vi "7_segment.vi"() -> ()   [LabVIEW 2019]
panel:
  in  "Numeric":i32
  out "F":bool
  out "E":bool
  out "C":bool
  out "B":bool
  out "D":bool
  out "G":bool
  out "A":bool
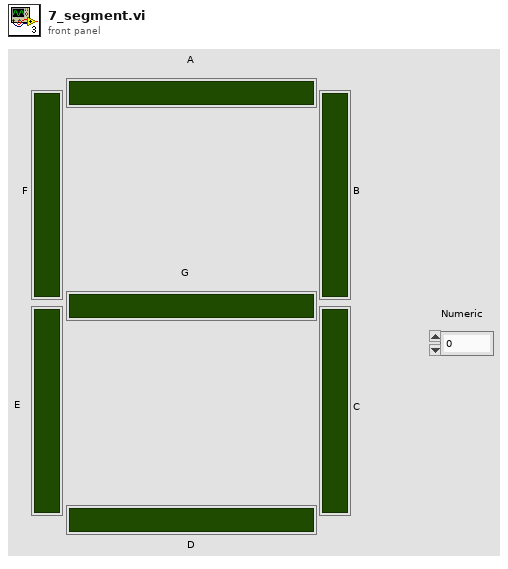
[diagram p1: front panel]
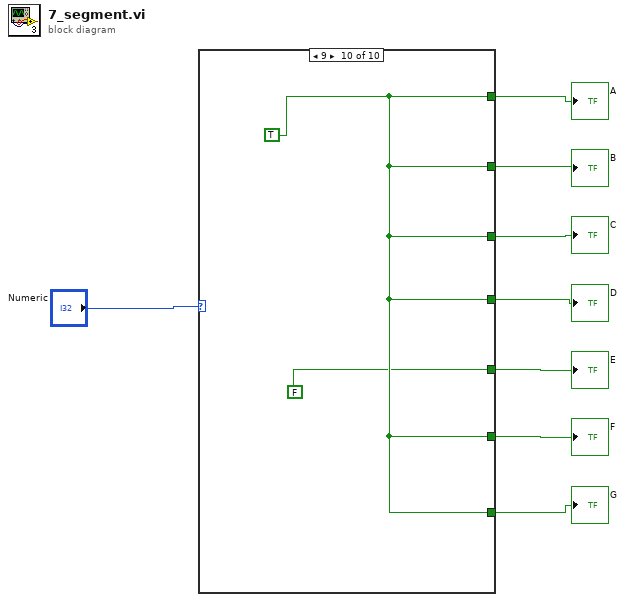
[diagram p0: block diagram]
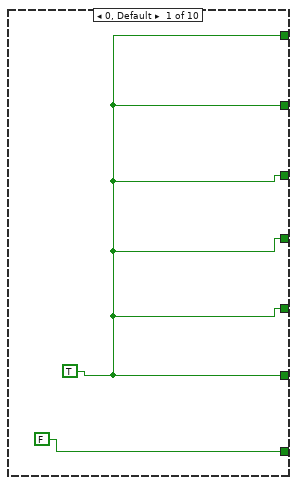
[diagram p2: hidden frame]
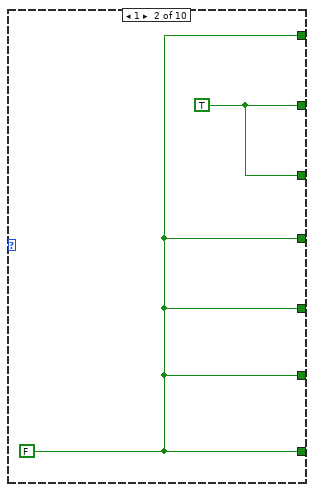
[diagram p3: hidden frame]
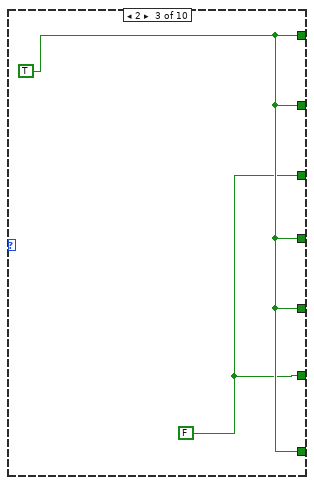
[diagram p4: hidden frame]
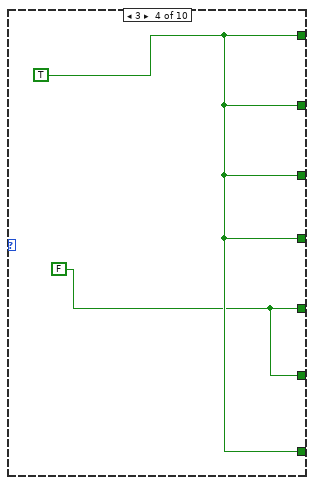
[diagram p5: hidden frame]
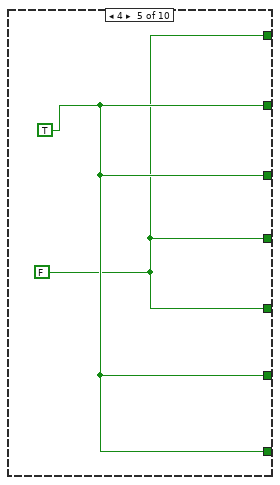
[diagram p6: hidden frame]
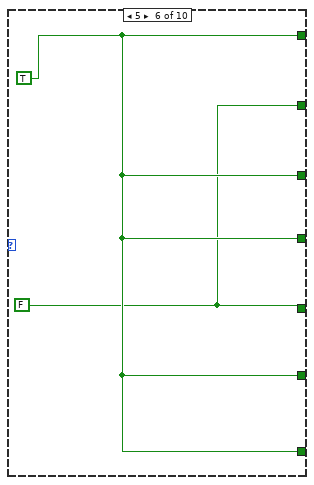
[diagram p7: hidden frame]
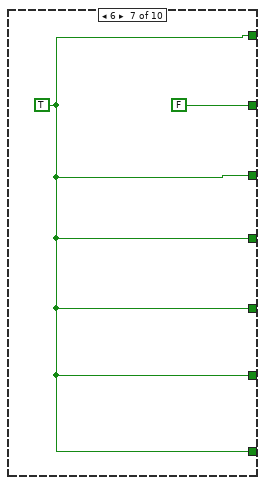
[diagram p8: hidden frame]
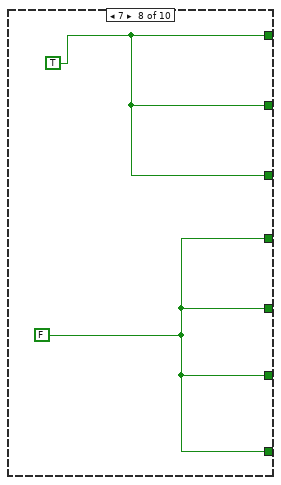
[diagram p9: hidden frame]
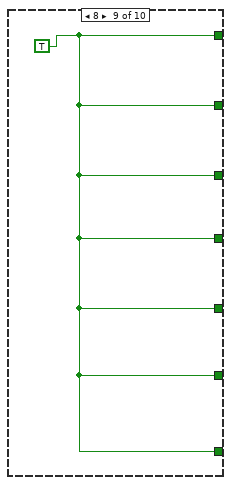
[diagram p10: hidden frame]
diagram:
  n1 = case shown="9" "Numeric" {
    tunnel: [w10 w11 w14 w16 w17 w20 w21 w24 w25 w27] -> w7
    tunnel: [w10 w12 w14 w16 w18 w19 FALSE w24 w25 w27] -> w6
    tunnel: [w10 w12 w13 w16 w18 w20 w21 w24 w25 w27] -> w5
    tunnel: [FALSE w11 w14 w16 w18 w20 w21 w23 w25 w27] -> w4
    tunnel: [w10 w11 w13 w15 w18 w20 w21 w23 w25 w27] -> w3
    tunnel: [w10 w11 w14 w15 w17 w19 w21 w23 w25 FALSE] -> w2
    tunnel: [w10 w11 w14 w16 w17 w20 w21 w23 w25 w27] -> w1
    frame 0, Default {
      w10 = TRUE
    }
    frame 1 {
      w12 = TRUE
      w11 = FALSE
    }
    frame 2 {
      w13 = FALSE
      w14 = TRUE
    }
    frame 3 {
      w15 = FALSE
      w16 = TRUE
    }
    frame 4 {
      w17 = FALSE
      w18 = TRUE
    }
    frame 5 {
      w19 = FALSE
      w20 = TRUE
    }
    frame 6 {
      w21 = TRUE
    }
    frame 7 {
      w23 = FALSE
      w24 = TRUE
    }
    frame 8 {
      w25 = TRUE
    }
    frame 9 {
      w27 = TRUE
    }
  }
  "A" <- w7
  "G" <- w4
  "D" <- w1
  "B" <- w6
  "C" <- w5
  "E" <- w2
  "F" <- w3
